vi "ClimbNetwork.vi"(8 "error in (no error)":errorcluster) -> (0 "error out":errorcluster)   [LabVIEW 2023]
uses:
  ClimbGlobal.vi
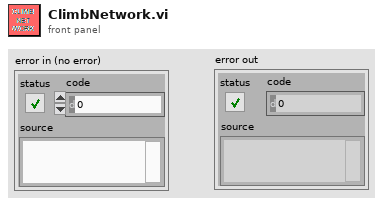
[diagram p1: front panel]
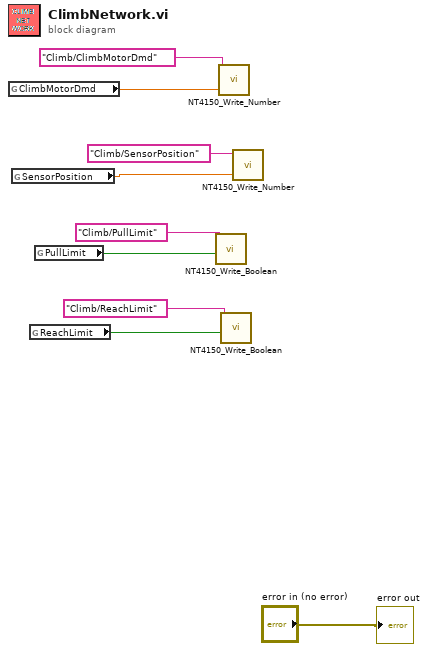
[diagram p0: block diagram]
diagram:
  n1 = global read "ClimbGlobal.vi" "ClimbMotorDmd"() -> (w8:dbl)
  n2 = global read "ClimbGlobal.vi" "SensorPosition"() -> (w7:dbl)
  n3 = global read "ClimbGlobal.vi" "ReachLimit"() -> (w5:bool)
  n4 = global read "ClimbGlobal.vi" "PullLimit"() -> (w6:bool)
  n5 = call "NT4150_Write_Boolean.vi"("value"=w6, "name"="Climb/PullLimit") -> ()  [unwired: 9 in, 1 out]
  n6 = call "NT4150_Write_Number.vi"("value"=w8, "name"="Climb/ClimbMotorDmd") -> ()  [unwired: 9 in, 1 out]
  n7 = call "NT4150_Write_Boolean.vi"("value"=w5, "name"="Climb/ReachLimit") -> ()  [unwired: 9 in, 1 out]
  n8 = call "NT4150_Write_Number.vi"("value"=w7, "name"="Climb/SensorPosition") -> ()  [unwired: 9 in, 1 out]
  "error out" <- "error in (no error)"
